vi "runStraight.vi"(11 "Distance In":dbl) -> ()   [LabVIEW 2015]
uses:
  Robot Global Data.vi
  <vilib>/addons/control/pid/pid.llb/PID (DBL).vi
  <vilib>/addons/control/pid/NI_PID_pid.lvlib
panel:
  in  "Distance In 2":dbl
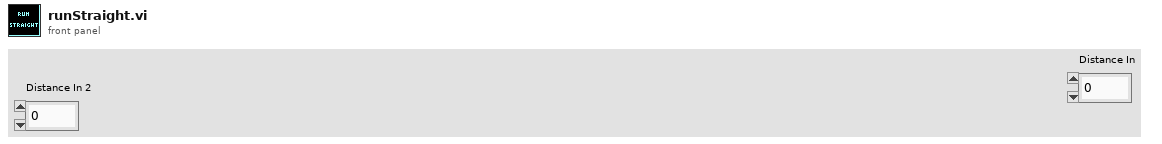
[diagram p1: front panel]
types:
  T1 = typedef "WPI_GyroDevRef.ctl" = cluster{"DevStatus":errorcluster, "Analog Channel":T2, "Offset":dbl, "Gain (VoltsPerDegree/Second)":dbl, "Gyro Type":enum16{"Analog", "XRS450"}, "Handle":i32, "SPI Bus":T3, "Device Found":bool, "Sample Rate":dbl, "Calibrate On Open":bool}
  T2 = typedef "FPGA_AIChannel.ctl" = enum8{"AI 0", "AI 1", "AI 2", "AI 3", "AI MXP 0", "AI MXP 1", "AI MXP 2", "AI MXP 3", "Invalid"}
  T3 = typedef "spi_bus.ctl" = enum16{"SPI On-Board, CS0", "SPI On-Board, CS1", "SPI On-Board, CS2", "SPI On-Board, CS3", "SPI MXP", "Invalid"}
  T4 = typedef "WPI_EncoderDevRef.ctl" = cluster{"DevStatus":errorcluster, "EncoderIndex":T5, "CounterIndex":T6, "DistancePerCount":dbl, "Decoding Type":T7}
  T5 = typedef "FPGA_EncoderIdx.ctl" = enum8{"Enc 0", "Enc 1", "Enc 2", "Enc 3", "Enc 4", "Enc 5", "Enc 6", "Enc 7", "Invalid"}
  T6 = typedef "FPGA_CounterCtrSystemIndex.ctl" = enum8{"Ctr 0", "Ctr 1", "Ctr 2", "Ctr 3", "Ctr 4", "Ctr 5", "Ctr 6", "Ctr 7", "Invalid"}
  T7 = typedef "WPI_EncoderType.ctl" = enum16{"1x", "2x", "4x"}
  T8 = cluster{"proportional gain (Kc)":dbl, "integral time (Ti, min)":dbl, "derivative time (Td, min)":dbl}
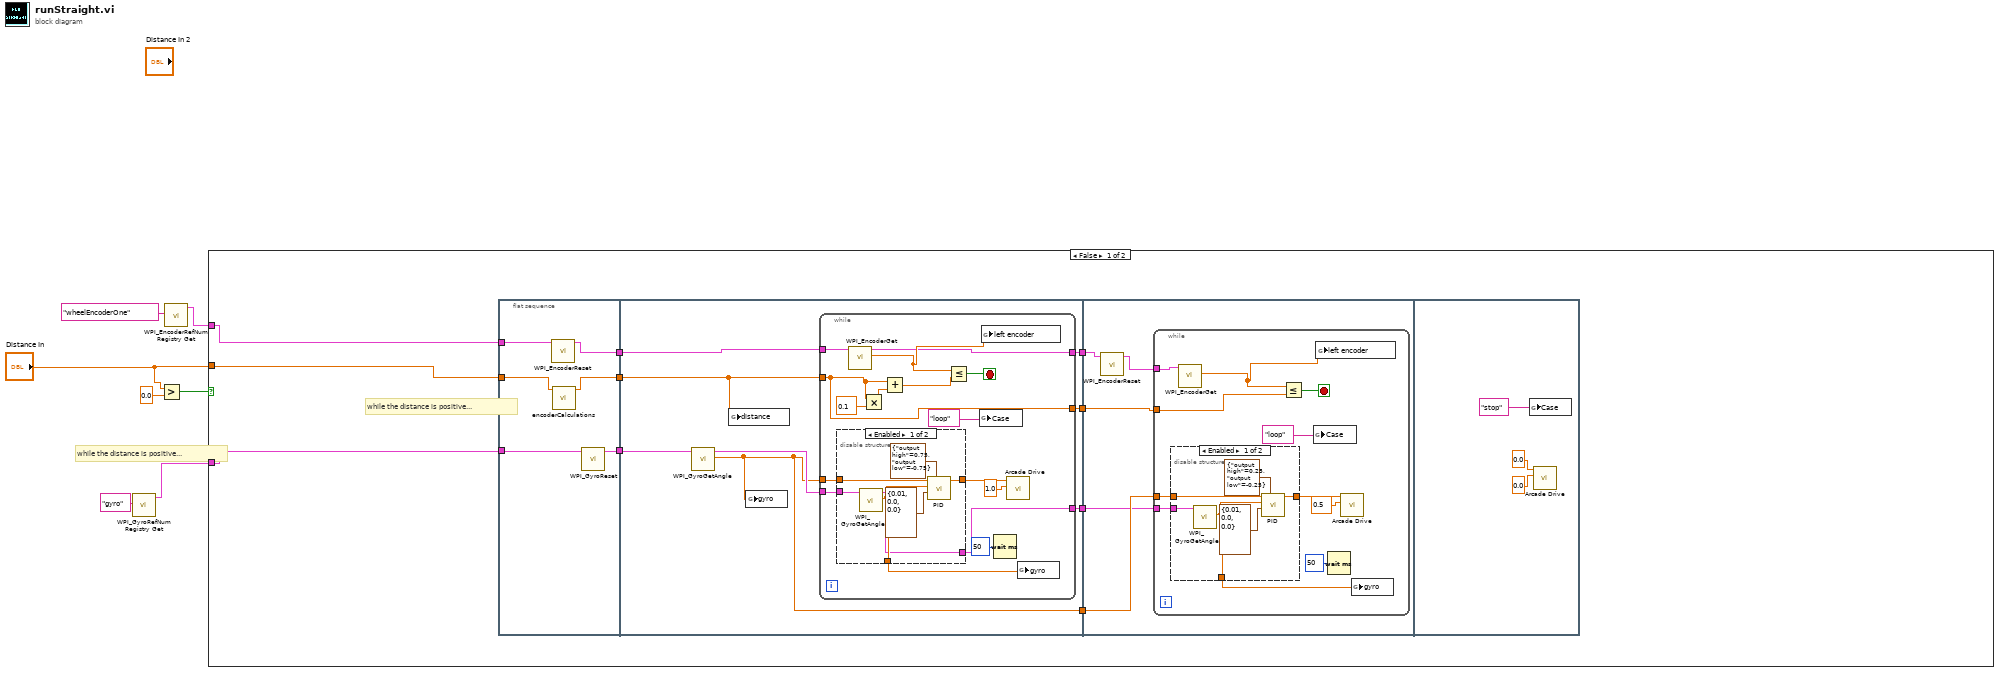
[diagram p0: block diagram]
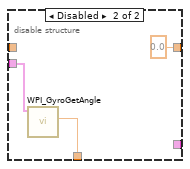
[diagram p2: hidden frame]
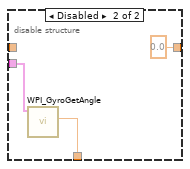
[diagram p3: hidden frame]
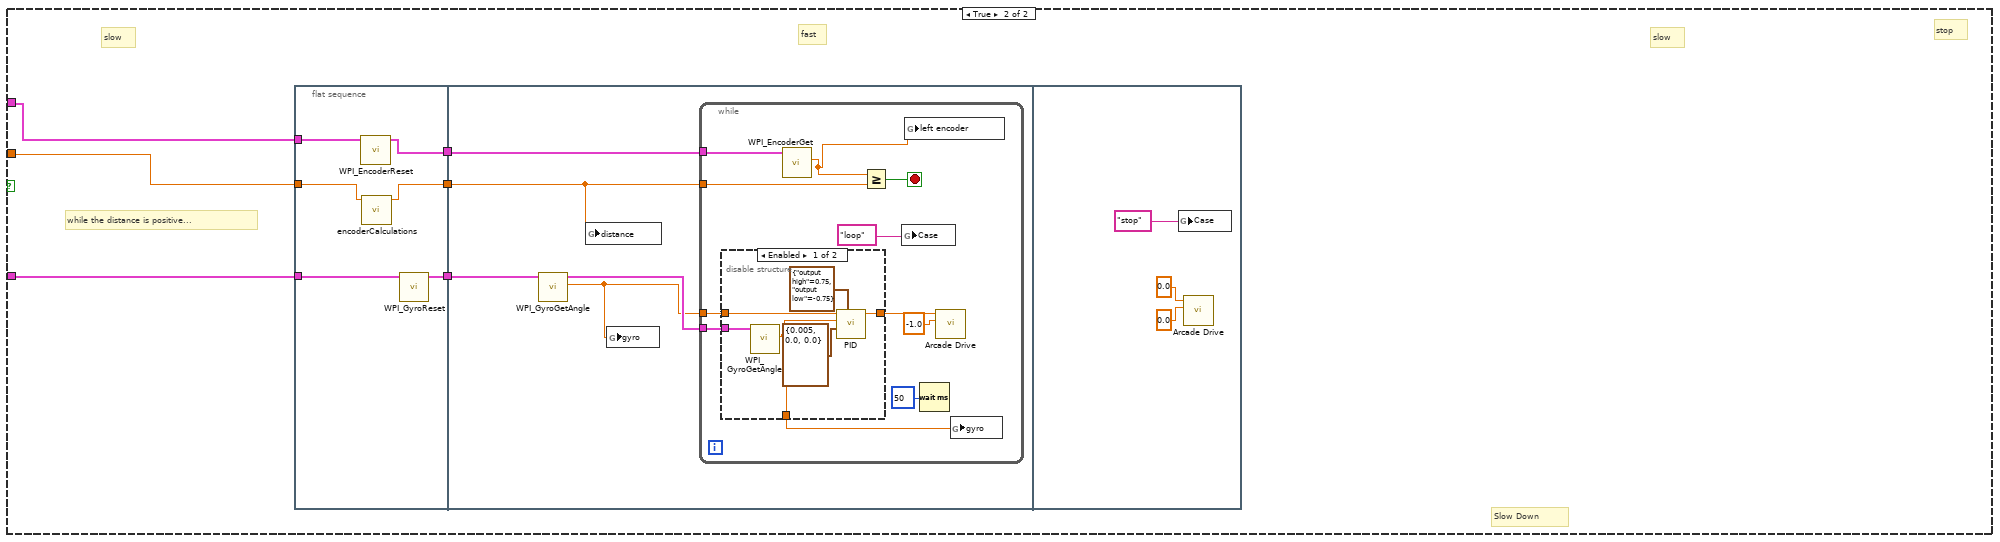
[diagram p4: hidden frame]
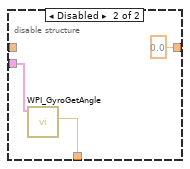
[diagram p5: hidden frame]
diagram:
  # "while the distance is positive..."
  n1 = call <vilib>:"WPI_GyroRefNum Registry Get.vi"("refnum name"="gyro") -> ("GyroDevRef"=w1:T1)  [unwired: 9 in, 1 out]
  n2 = Greater?(x="Distance In", y=0.0) -> (0:w6:bool)
  n3 = call <vilib>:"WPI_EncoderRefNum Registry Get.vi"("refnum name"="wheelEncoderOne") -> ("EncoderDevRef"=w3:T4)  [unwired: 9 in, 1 out]
  n4 = case shown="False" w6 {
    tunnel: "Distance In" -> [w13 w89]
    tunnel: w3 -> [w14 w87]
    tunnel: w1 -> [w12 w88]
    frame False {
      # "while the distance is positive..."
      n5 = flat-sequence {
        tunnel: w13 -> [w22]
        tunnel: [w21] -> w17
        tunnel: [w23] -> w16
        tunnel: w12 -> [w20]
        tunnel: w14 -> [w19]
        tunnel: [w18] -> w15
        tunnel: w17 -> [w29]
        tunnel: w16 -> [w30]
        tunnel: w15 -> [w28]
        tunnel: [w27] -> w11
        tunnel: [w26] -> w10
        tunnel: [w25] -> w9
        tunnel: [w24] -> w8
        tunnel: w11 -> [w62]
        tunnel: w10 -> [w60]
        tunnel: w9 -> [w59]
        tunnel: w8 -> [w58]
        frame #0 {
          n6 = call <vilib>:"WPI_EncoderReset.vi"("EncoderDevRef"=w19) -> ("EncoderDevRef"=w18:T4)  [unwired: 9 in, 1 out]
          n7 = call "encoderCalculations.vi"("Left Distance In"=w22) -> ("Left Ticks"=w21:dbl)  [unwired: 9 in, 1 out]
          n8 = call <vilib>:"WPI_GyroReset.vi"("GyroDevRef"=w20) -> ("GyroDevRef"=w23:T1)  [unwired: 9 in, 1 out]
        }
        frame #1 {
          n9 = call <vilib>:"WPI_GyroGetAngle.vi"("GyroDevRef"=w30) -> ("Angle"=w25:dbl, "GyroDevRef"=w31:T1)  [unwired: 6 in, 3 out]
          n10 = global write "Robot Global Data.vi" "distance"(w29) -> ()
          n11 = global write "Robot Global Data.vi" "gyro"(w25) -> ()
          n12 = while {
            tunnel: w29 -> [w33]
            tunnel: w25 -> [w46]
            tunnel: w31 -> [w45]
            tunnel: w28 -> [w38]
            tunnel: [w37] -> w27
            tunnel: [w33] -> w26
            tunnel: [w32] -> w24
            stop <- w47 stop-if-true
            n13 = disable-structure shown="Enabled" {
              disable-tunnel: w46 -> [w52 _]
              disable-tunnel: w45 -> [w51 w55]
              disable-tunnel: [w50 0.0 ("x")] -> w44
              disable-tunnel: [w49 w56] -> w39
              disable-tunnel: [w48 _] -> w32
              frame Enabled {
                n14 = call <vilib>:"WPI_GyroGetAngle.vi"("GyroDevRef"=w51) -> ("Angle"=w49:dbl, "GyroDevRef"=w48:T1)  [unwired: 6 in, 3 out]
                n15 = call-poly <vilib>:"PID.vi"("output range"=cluster{"output high":dbl, "output low":dbl} {"output high"=0.75, "output low"=-0.75}, "PID gains"=T8 {"proportional gain (Kc)"=0.01, "integral time (Ti, min)"=0.0, "derivative time (Td, min)"=0.0}, "process variable"=w49, "setpoint"=w52) -> ("output"=w50:dbl)  [unwired: 6 in, 1 out]
              }
              frame Disabled {
                n16 = call <vilib>:"WPI_GyroGetAngle.vi"("GyroDevRef"=w55) -> ("Angle"=w56:dbl)  [unwired: 6 in, 4 out]
              }
            }
            n17 = call <vilib>:"WPI_EncoderGet.vi"("EncoderDevRef"=w38) -> ("Distance"=w40:dbl, "EncoderDevRef"=w37:T4)  [unwired: 5 in, 4 out]
            n18 = Multiply(x=w33, y=0.1) -> (x*y=w35:dbl)
            n19 = Add(x=w33, y=w35) -> (x+y=w34:dbl)
            n20 = Less Or Equal?(x=w40, y=w34) -> (x <= y?=w47:bool)
            n21 = global write "Robot Global Data.vi" "Case"("loop") -> ()
            n22 = global write "Robot Global Data.vi" "left encoder"(w40) -> ()
            n23 = Wait (ms)(milliseconds to wait=u32 50) -> ()  [unwired: 1 out]
            n24 = call "Arcade Drive.vi"("y"=1.0, "x"=w44) -> ()  [unwired: 10 in]
            n25 = global write "Robot Global Data.vi" "gyro"(w39) -> ()
          }
        }
        frame #2 {
          n26 = call <vilib>:"WPI_EncoderReset.vi"("EncoderDevRef"=w62) -> ("EncoderDevRef"=w61:T4)  [unwired: 9 in, 1 out]
          n27 = while {
            tunnel: w60 -> [w73]
            tunnel: w59 -> [w71]
            tunnel: w58 -> [w70]
            tunnel: w61 -> [w63]
            stop <- w72 stop-if-true
            n28 = disable-structure shown="Enabled" {
              disable-tunnel: w71 -> [w77 _]
              disable-tunnel: w70 -> [w76 w80]
              disable-tunnel: [w75 0.0 ("x")] -> w69
              disable-tunnel: [w74 w81] -> w64
              frame Enabled {
                n29 = call <vilib>:"WPI_GyroGetAngle.vi"("GyroDevRef"=w76) -> ("Angle"=w74:dbl)  [unwired: 6 in, 4 out]
                n30 = call-poly <vilib>:"PID.vi"("output range"=cluster{"output high":dbl, "output low":dbl} {"output high"=0.25, "output low"=-0.25}, "PID gains"=T8 {"proportional gain (Kc)"=0.01, "integral time (Ti, min)"=0.0, "derivative time (Td, min)"=0.0}, "process variable"=w74, "setpoint"=w77) -> ("output"=w75:dbl)  [unwired: 6 in, 1 out]
              }
              frame Disabled {
                n31 = call <vilib>:"WPI_GyroGetAngle.vi"("GyroDevRef"=w80) -> ("Angle"=w81:dbl)  [unwired: 6 in, 4 out]
              }
            }
            n32 = call <vilib>:"WPI_EncoderGet.vi"("EncoderDevRef"=w63) -> ("Distance"=w65:dbl)  [unwired: 5 in, 5 out]
            n33 = Less Or Equal?(x=w65, y=w73) -> (x <= y?=w72:bool)
            n34 = global write "Robot Global Data.vi" "Case"("loop") -> ()
            n35 = global write "Robot Global Data.vi" "left encoder"(w65) -> ()
            n36 = Wait (ms)(milliseconds to wait=u32 50) -> ()  [unwired: 1 out]
            n37 = call "Arcade Drive.vi"("y"=0.5, "x"=w69) -> ()  [unwired: 10 in]
            n38 = global write "Robot Global Data.vi" "gyro"(w64) -> ()
          }
        }
        frame #3 {
          n39 = global write "Robot Global Data.vi" "Case"("stop") -> ()
          n40 = call "Arcade Drive.vi"("y"=0.0, "x"=0.0) -> ()  [unwired: 10 in]
        }
      }
    }
    frame True {
      # "stop"
      # "slow"
      # "fast"
      # "slow"
      # "while the distance is positive..."
      # "Slow Down"
      n41 = flat-sequence {
        tunnel: w89 -> [w96]
        tunnel: [w95] -> w91
        tunnel: [w97] -> w90
        tunnel: w88 -> [w94]
        tunnel: w87 -> [w93]
        tunnel: [w92] -> w86
        tunnel: w91 -> [w99]
        tunnel: w90 -> [w100]
        tunnel: w86 -> [w98]
        frame #0 {
          n42 = call <vilib>:"WPI_EncoderReset.vi"("EncoderDevRef"=w93) -> ("EncoderDevRef"=w92:T4)  [unwired: 9 in, 1 out]
          n43 = call "encoderCalculations.vi"("Left Distance In"=w96) -> ("Left Ticks"=w95:dbl)  [unwired: 9 in, 1 out]
          n44 = call <vilib>:"WPI_GyroReset.vi"("GyroDevRef"=w94) -> ("GyroDevRef"=w97:T1)  [unwired: 9 in, 1 out]
        }
        frame #1 {
          n45 = call <vilib>:"WPI_GyroGetAngle.vi"("GyroDevRef"=w100) -> ("Angle"=w101:dbl, "GyroDevRef"=w102:T1)  [unwired: 6 in, 3 out]
          n46 = global write "Robot Global Data.vi" "distance"(w99) -> ()
          n47 = global write "Robot Global Data.vi" "gyro"(w101) -> ()
          n48 = while {
            tunnel: w99 -> [w113]
            tunnel: w101 -> [w111]
            tunnel: w102 -> [w110]
            tunnel: w98 -> [w103]
            stop <- w112 stop-if-true
            n49 = disable-structure shown="Enabled" {
              disable-tunnel: w111 -> [w117 _]
              disable-tunnel: w110 -> [w116 w120]
              disable-tunnel: [w115 0.0 ("x")] -> w109
              disable-tunnel: [w114 w121] -> w104
              frame Enabled {
                n50 = call <vilib>:"WPI_GyroGetAngle.vi"("GyroDevRef"=w116) -> ("Angle"=w114:dbl)  [unwired: 6 in, 4 out]
                n51 = call-poly <vilib>:"PID.vi"("output range"=cluster{"output high":dbl, "output low":dbl} {"output high"=0.75, "output low"=-0.75}, "PID gains"=T8 {"proportional gain (Kc)"=0.005, "integral time (Ti, min)"=0.0, "derivative time (Td, min)"=0.0}, "process variable"=w114, "setpoint"=w117) -> ("output"=w115:dbl)  [unwired: 6 in, 1 out]
              }
              frame Disabled {
                n52 = call <vilib>:"WPI_GyroGetAngle.vi"("GyroDevRef"=w120) -> ("Angle"=w121:dbl)  [unwired: 6 in, 4 out]
              }
            }
            n53 = call <vilib>:"WPI_EncoderGet.vi"("EncoderDevRef"=w103) -> ("Distance"=w105:dbl)  [unwired: 5 in, 5 out]
            n54 = Greater Or Equal?(x=w105, y=w113) -> (x >= y?=w112:bool)
            n55 = global write "Robot Global Data.vi" "Case"("loop") -> ()
            n56 = global write "Robot Global Data.vi" "left encoder"(w105) -> ()
            n57 = Wait (ms)(milliseconds to wait=u32 50) -> ()  [unwired: 1 out]
            n58 = call "Arcade Drive.vi"("y"=-1.0, "x"=w109) -> ()  [unwired: 10 in]
            n59 = global write "Robot Global Data.vi" "gyro"(w104) -> ()
          }
        }
        frame #2 {
          n60 = global write "Robot Global Data.vi" "Case"("stop") -> ()
          n61 = call "Arcade Drive.vi"("y"=0.0, "x"=0.0) -> ()  [unwired: 10 in]
        }
      }
    }
  }
